vi "Linear_Track_Filter-4.vi"(6 "[IN] Max angle":dbl, 7 "[IN] % track linearity":i32, 8 "error IN":errorcluster, 11 "[IN] Tracks w/t Problems":T2(array[cluster])) -> (0 "error OUT":errorcluster, 1 "[OUT] Nonlinear Tracks":T1(array[cluster]), 3 "[OUT] Linear Tracks (Filtered)":T2(array[cluster]))   [LabVIEW 2013]
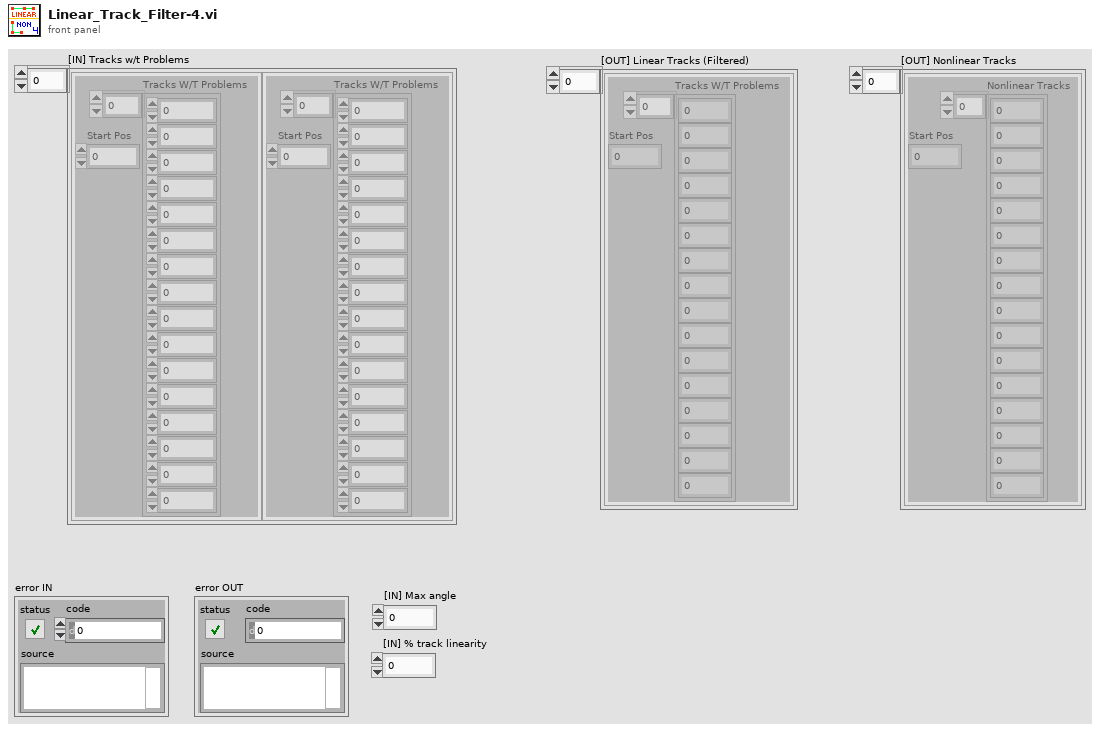
[diagram p1: front panel]
types:
  T1 = cluster{"Nonlinear Tracks":dbl[], "Start Pos":i32}[]
  T2 = cluster{"Tracks W/T Problems":dbl[], "Start Pos":i32}[]
  T3 = cluster{"Nonlinear Tracks":dbl[], "Start Pos":i32}
  T4 = cluster{"Tracks W/T Problems":dbl[], "Start Pos":i32}
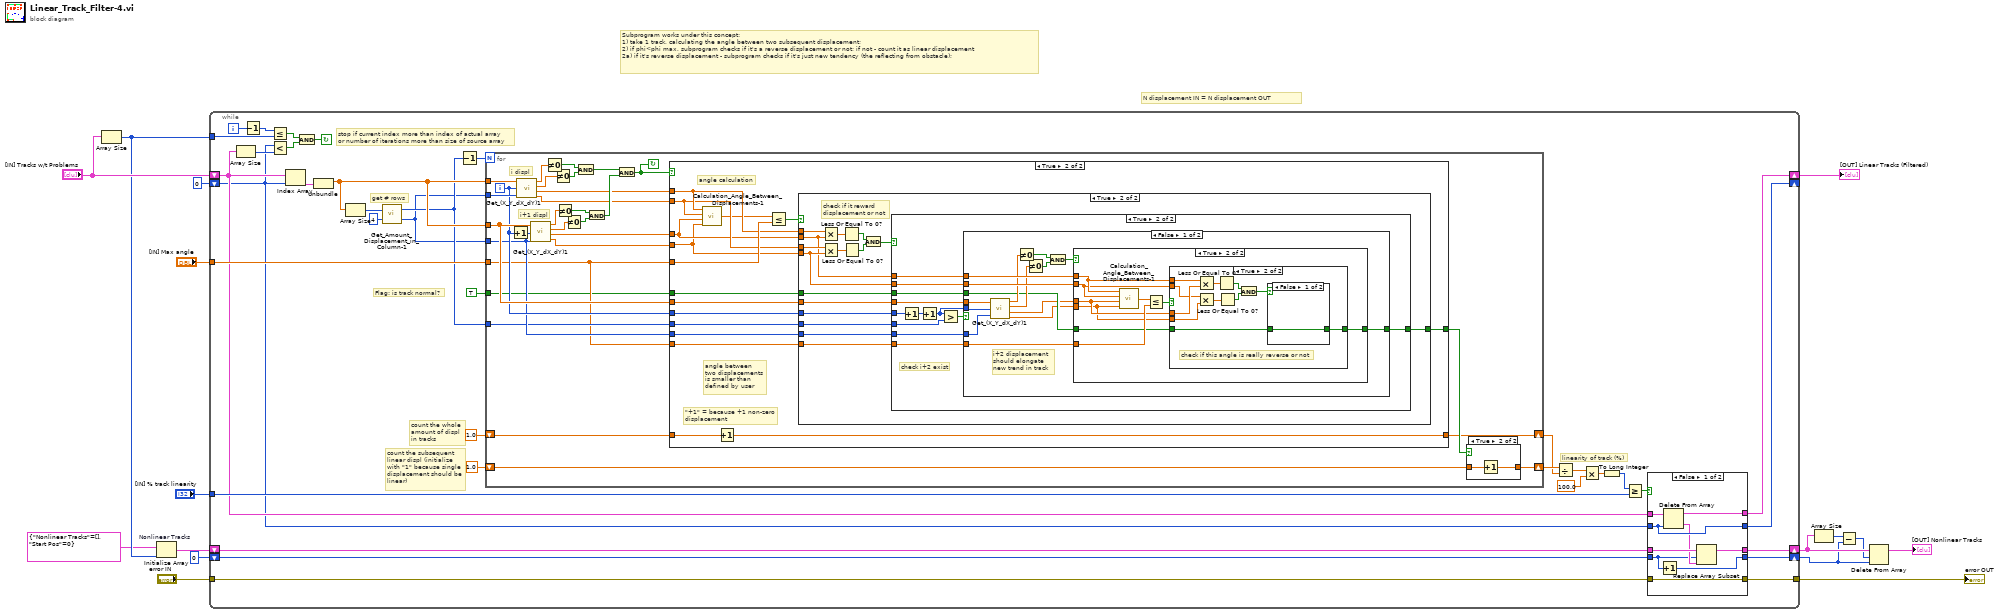
[diagram p0: block diagram]
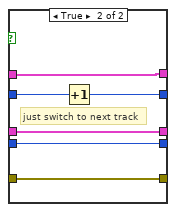
[diagram p2: hidden frame]
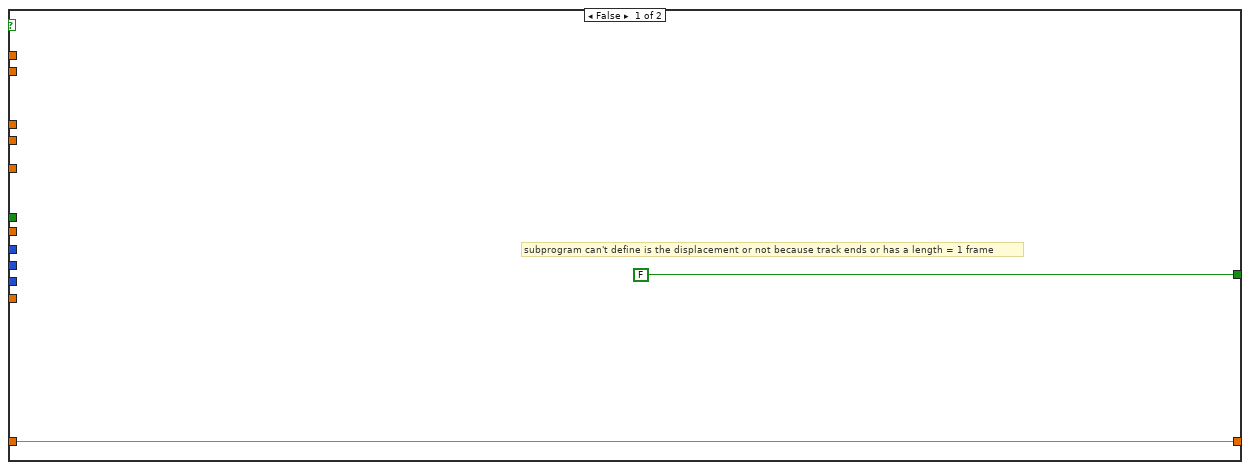
[diagram p4: hidden frame]
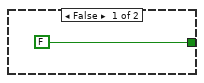
[diagram p5: hidden frame]
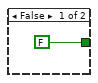
[diagram p7: hidden frame]
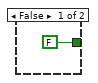
[diagram p8: hidden frame]
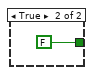
[diagram p9: hidden frame]
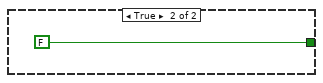
[diagram p10: hidden frame]
diagram:
  # "N displacement IN = N displacement OUT"
  # "Subprogram works under this concept:\n1) take 1 track, calculating the angle between two subsequent displacement; \n2) if phi<phi max, subprogram checks if it's a reverse displacement or not; if not - count it as linear displacement\n2a) if it's reverse displacement - subprogram checks if it's just new tendency (the reflecting from obstacle);"
  n1 = Array Size(array="[IN] Tracks w/t Problems") -> (size(s)=w10:i32)
  n2 = Initialize Array "Nonlinear Tracks"(T3 {"Nonlinear Tracks"=[], "Start Pos"=0} ("element"), w10) -> (w8:T1)
  n3 = while {
    tunnel: "[IN] Max angle" -> [w52]
    tunnel: "error IN" -> [w18]
    tunnel: [w17] -> w14
    tunnel: "[IN] % track linearity" -> [w40]
    shift-right: [w24] -> w6
    shift-left: "[IN] Tracks w/t Problems" -> [w28]
    tunnel: w10 -> [w33]
    shift-right: [w23] -> _
    shift-left: 0 -> [w25]
    shift-right: [w20] -> w5
    shift-left: w8 -> [w22]
    shift-right: [w19] -> w3
    shift-left: 0 -> [w21]
    i -> [w27]
    stop <- w29 continue-if-true
    # "stop if current index more than index of actual array \nor number of iterations more than size of source array"
    # "get # rows"
    # "linearity of track (%)"
    # "count the subsequent\nlinear displ (initialize \nwith \"1\" because single\ndisplacement should be\nlinear)"
    # "count the whole\namount of displ\nin tracks"
    # "Flag: is track normal?"
    n4 = Array Size(array=w28) -> (size(s)=w31:i32)
    n5 = Decrement(x=w27) -> (x-1=w26:i32)
    n6 = Less Or Equal?(x=w26, y=w33) -> (x <= y?=w32:bool)
    n7 = Less?(x=w25, y=w31) -> (x < y?=w30:bool)
    n8 = Index Array(array=w28, index=w25) -> (element=w39:T4)
    n9 = And(x=w32, y=w30) -> (x .and. y?=w29:bool)
    n10 = Unbundle(w39) -> ("Tracks W/T Problems"=w37:dbl[])  [unwired: 1 out]
    n11 = Array Size(array=w37) -> (size(s)=w36:i32)
    n12 = call "Get_Amount_Displacement_in_Column-1.vi"("multiplier"=4, "# Rows"=w36) -> ("multiplier out"=w34:i32, "Displ amount"=w35:i32)
    n13 = Decrement(x=w35) -> (x-1=w51:i32)
    n14 = for {
      N: w51 -> [_]
      tunnel: w37 -> [w96]
      tunnel: w34 -> [w90]
      tunnel: w37 -> [w82]
      tunnel: w34 -> [w80]
      tunnel: w52 -> [w75]
      tunnel: w35 -> [w76]
      tunnel: TRUE -> [w74]
      shift-right: [w70] -> w46
      shift-left: 1.0 -> [w71]
      shift-right: [w68] -> w47
      shift-left: 1.0 -> [w69]
      i -> [w81]
      stop <- w73 continue-if-true
      # "i+1 displ"
      # "i displ"
      n15 = Increment(x=w81) -> (x+1=w91:i32)
      n16 = call "Get_(X_Y_dX_dY)1.vi"("(X,Y,dX,dY)"=w96, "index"=w81, "multiplier"=w90) -> ("X"=w95:dbl, "Y"=w94:dbl, "dX"=w79:dbl, "dY"=w83:dbl)
      n17 = call "Get_(X_Y_dX_dY)1.vi"("(X,Y,dX,dY)"=w82, "index"=w91, "multiplier"=w80) -> ("X"=w87:dbl, "Y"=w86:dbl, "dX"=w78:dbl, "dY"=w77:dbl)
      n18 = Not Equal To 0?(x=w95) -> (x != 0?=w92:bool)
      n19 = Not Equal To 0?(x=w94) -> (x != 0?=w93:bool)
      n20 = Not Equal To 0?(x=w87) -> (x != 0?=w88:bool)
      n21 = Not Equal To 0?(x=w86) -> (x != 0?=w89:bool)
      n22 = And(x=w92, y=w93) -> (x .and. y?=w85:bool)
      n23 = And(x=w88, y=w89) -> (x .and. y?=w84:bool)
      n24 = And(x=w85, y=w84) -> (x .and. y?=w73:bool)
      n25 = case shown="True" w73 {
        tunnel: w83 -> [_ w105]
        tunnel: w79 -> [_ w106]
        tunnel: w78 -> [_ w104]
        tunnel: w77 -> [_ w103]
        tunnel: w75 -> [_ w117]
        tunnel: w74 -> [_ w115]
        tunnel: [FALSE w114] -> w72
        tunnel: w82 -> [_ w113]
        tunnel: w81 -> [_ w112]
        tunnel: w80 -> [_ w111]
        tunnel: w76 -> [_ w110]
        tunnel: w75 -> [_ w109]
        tunnel: w71 -> [w101 w107]
        tunnel: [w101 w108] -> w70
        frame False {
          # "subprogram can't define is the displacement or not because track ends or has a length = 1 frame"
        }
        frame True {
          # "\"+1\" = because +1 non-zero\ndisplacement"
          # "angle calculation"
          # "angle between\ntwo displacements\nis smaller than \ndefined by user"
          n26 = call "Calculation_Angle_Between_Displacements-1.vi"("dY 2"=w103, "dX 2"=w104, "dY 1"=w105, "dX 1"=w106) -> ("angle in degrees"=w102:dbl)
          n27 = Increment(x=w107) -> (x+1=w108:dbl)
          n28 = Less Or Equal?(x=w102, y=w117) -> (x <= y?=w116:bool)
          n29 = case shown="True" w116 {
            tunnel: w104 -> [_ w119]
            tunnel: w103 -> [_ w121]
            tunnel: w106 -> [_ w134]
            tunnel: w105 -> [_ w122]
            tunnel: w115 -> [_ w128]
            tunnel: [FALSE w127] -> w114
            tunnel: w113 -> [_ w126]
            tunnel: w112 -> [_ w125]
            tunnel: w111 -> [_ w124]
            tunnel: w110 -> [_ w123]
            tunnel: w109 -> [_ w120]
            frame False {
            }
            frame True {
              # "check if it reward \ndisplacement or not"
              n30 = Multiply(x=w134, y=w119) -> (x*y=w133:dbl)
              n31 = Multiply(x=w122, y=w121) -> (x*y=w132:dbl)
              n32 = Less Or Equal To 0?(x=w133) -> (x <= 0?=w130:bool)
              n33 = Less Or Equal To 0?(x=w132) -> (x <= 0?=w131:bool)
              n34 = And(x=w130, y=w131) -> (x .and. y?=w129:bool)
              n35 = case shown="True" w129 {
                tunnel: w128 -> [w135 w143]
                tunnel: [w135 w142] -> w127
                tunnel: w126 -> [_ w141]
                tunnel: w125 -> [_ w147]
                tunnel: w124 -> [_ w139]
                tunnel: w123 -> [_ w145]
                tunnel: w119 -> [_ w138]
                tunnel: w121 -> [_ w137]
                tunnel: w120 -> [_ w136]
                frame False {
                }
                frame True {
                  # "check i+2 exist"
                  n36 = Increment(x=w147) -> (x+1=w146:i32)
                  n37 = Increment(x=w146) -> (x+1=w140:i32)
                  n38 = Greater?(x=w140, y=w145) -> (0:w144:bool)
                  n39 = case shown="False" w144 {
                    tunnel: w143 -> [w152 _]
                    tunnel: [w148 FALSE] -> w142
                    tunnel: w141 -> [w159 _]
                    tunnel: w140 -> [w158 _]
                    tunnel: w139 -> [w157 _]
                    tunnel: w138 -> [w156 _]
                    tunnel: w137 -> [w155 _]
                    tunnel: w136 -> [w151 _]
                    frame False {
                      # "i+2 displacement \nshould elongate\nnew trend in track"
                      n40 = call "Get_(X_Y_dX_dY)1.vi"("(X,Y,dX,dY)"=w159, "index"=w158, "multiplier"=w157) -> ("X"=w154:dbl, "Y"=w153:dbl, "dX"=w150:dbl, "dY"=w149:dbl)
                      n41 = Not Equal To 0?(x=w154) -> (x != 0?=w162:bool)
                      n42 = Not Equal To 0?(x=w153) -> (x != 0?=w161:bool)
                      n43 = And(x=w162, y=w161) -> (x .and. y?=w160:bool)
                      n44 = case shown="True" w160 {
                        tunnel: [FALSE w169] -> w148
                        tunnel: w156 -> [_ w168]
                        tunnel: w155 -> [_ w167]
                        tunnel: w150 -> [_ w166]
                        tunnel: w149 -> [_ w165]
                        tunnel: w152 -> [_ w170]
                        tunnel: w151 -> [_ w172]
                        frame False {
                        }
                        frame True {
                          n45 = call "Calculation_Angle_Between_Displacements-1.vi"("dY 2"=w165, "dX 2"=w166, "dY 1"=w167, "dX 1"=w168) -> ("angle in degrees"=w164:dbl)
                          n46 = Less Or Equal?(x=w164, y=w172) -> (x <= y?=w171:bool)
                          n47 = case shown="True" w171 {
                            tunnel: w168 -> [_ w180]
                            tunnel: w166 -> [_ w179]
                            tunnel: w165 -> [_ w178]
                            tunnel: w167 -> [_ w177]
                            tunnel: w170 -> [_ w175]
                            tunnel: [FALSE w174] -> w169
                            frame False {
                            }
                            frame True {
                              # "check if this angle is really reverse or not"
                              n48 = Multiply(x=w180, y=w179) -> (x*y=w184:dbl)
                              n49 = Multiply(x=w177, y=w178) -> (x*y=w183:dbl)
                              n50 = Less Or Equal To 0?(x=w184) -> (x <= 0?=w181:bool)
                              n51 = Less Or Equal To 0?(x=w183) -> (x <= 0?=w182:bool)
                              n52 = And(x=w181, y=w182) -> (x .and. y?=w176:bool)
                              n53 = case shown="False" w176 {
                                tunnel: w175 -> [w185 _]
                                tunnel: [w185 FALSE] -> w174
                                frame False {
                                }
                                frame True {
                                }
                              }
                            }
                          }
                        }
                      }
                    }
                    frame True {
                    }
                  }
                }
              }
            }
          }
        }
      }
      n54 = case shown="True" w72 {
        tunnel: w69 -> [w97 w99]
        tunnel: [w97 w98] -> w68
        frame False {
        }
        frame True {
          n55 = Increment(x=w99) -> (x+1=w98:dbl)
        }
      }
    }
    n56 = Divide(x=w47, y=w46) -> (x/y=w45:dbl)
    n57 = Multiply(x=w45, y=100.0) -> (x*y=w43:dbl)
    n58 = To Long Integer(number=w43) -> (32bit integer=w42:i32)
    n59 = Greater Or Equal?(x=w42, y=w40) -> (x >= y?=w41:bool)
    n60 = case shown="False" w41 {
      tunnel: w28 -> [w61 w67]
      tunnel: w25 -> [w59 w66]
      tunnel: [w60 w67] -> w24
      tunnel: [w59 w65] -> w23
      tunnel: w22 -> [w58 w64]
      tunnel: w21 -> [w55 w63]
      tunnel: [w56 w64] -> w20
      tunnel: [w54 w63] -> w19
      tunnel: w18 -> [w53 w62]
      tunnel: [w53 w62] -> w17
      frame False {
        n61 = Increment(x=w55) -> (x+1=w54:i32)
        n62 = Delete From Array(array=w61, index=w59) -> (deleted portion=w57:T4, array with subset deleted=w60:T2)  [unwired: 1 in]
        n63 = Replace Array Subset(array=w58, new element=w57, index=w55) -> (w56:T1)
      }
      frame True {
        # "just switch to next track"
        n64 = Increment(x=w66) -> (x+1=w65:i32)
      }
    }
  }
  "error OUT" <- w14
  "[OUT] Linear Tracks (Filtered)" <- w6
  n65 = Array Size(array=w5) -> (size(s)=w4:i32)
  n66 = Subtract(x=w4, y=w3) -> (x-y=w2:i32)
  n67 = Delete From Array(array=w5, length=w2, index=w3) -> (array with subset deleted=→"[OUT] Nonlinear Tracks":T1)  [unwired: 1 out]
